vi "Configure Average.vi"(5 "Filter Count (10)":i32=10, 6 "Filter Mode (0: Repeat)":i32(ring) items=["Repeat", "Moving"], 7 "Filter Type (1: Scalar)":i32(ring)=1 items=["None", "Scalar", "Advanced"], 8 "error in (no error)":errorcluster, 9 "Enable Average Filter (F: Disable)":bool, 10 "Measurement Function (0: Voltage)":i32(ring) items=["Voltage", "Current", "Resistance", "Charge"], 11 "VISA resource name":refnum<visa-resource-name>) -> (0 "error out":errorcluster, 3 "VISA resource name out":refnum<visa-resource-name>)   [LabVIEW 2019, in "Keithley 6517.lvlib"]
doc: "Configures the average settings for the measurement functions (Voltage, Current, Resistance and Charge).\n\nNote:\nThe specified measurement should be enabled from <b>Configure Measurement Function.vi</b>.\n\nThis VI is <B>NOT</B> compatible with model <B>6514</B>."
uses:
  Keithley 6517.lvlib
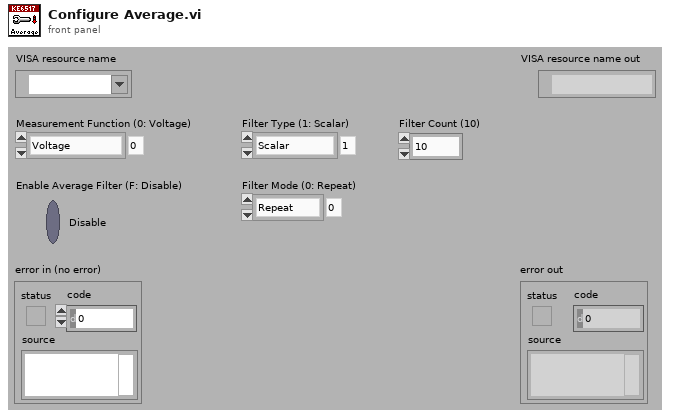
[diagram p1: front panel]
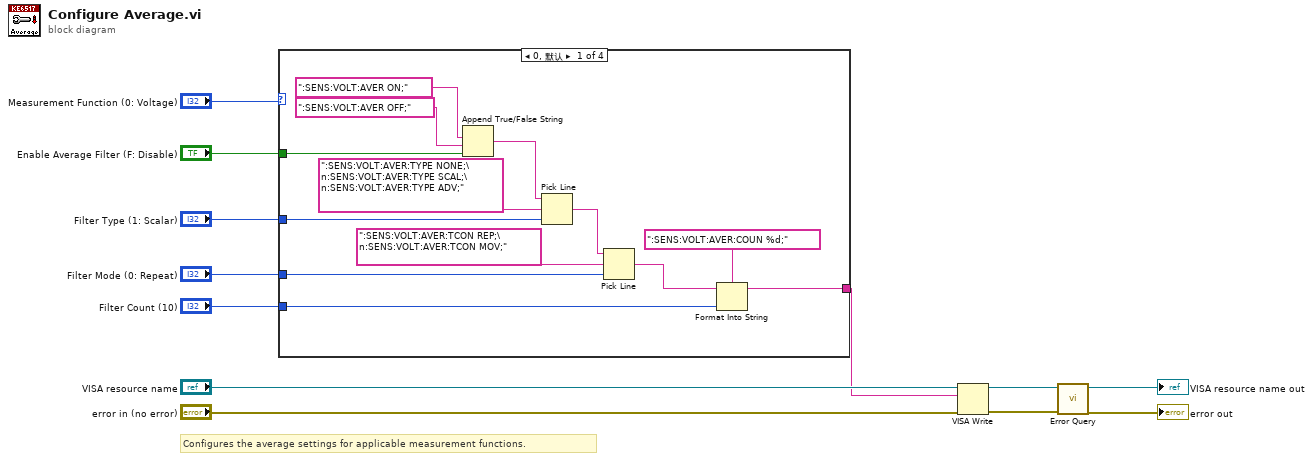
[diagram p0: block diagram]
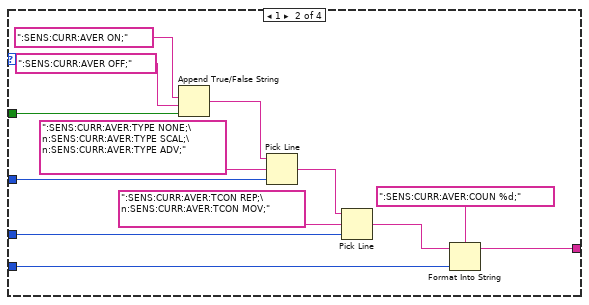
[diagram p2: hidden frame]
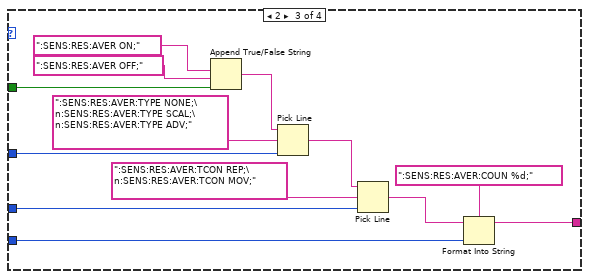
[diagram p3: hidden frame]
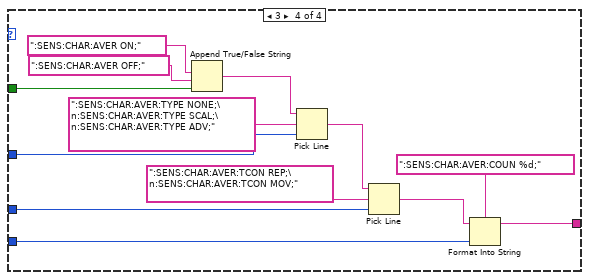
[diagram p4: hidden frame]
diagram:
  # "Configures the average settings for applicable measurement functions."
  n1 = case shown="0, 默认" "Measurement Function (0: Voltage)" {
    tunnel: "Enable Average Filter (F: Disable)" -> [w22 w35 w48 w61]
    tunnel: "Filter Type (1: Scalar)" -> [w19 w32 w45 w57]
    tunnel: "Filter Mode (0: Repeat)" -> [w16 w29 w44 w54]
    tunnel: "Filter Count (10)" -> [w15 w28 w40 w53]
    tunnel: [w13 w26 w39 w52] -> w3
    frame 0, Default {
      n2 = Append True/False String(1:w22, 2:":SENS:VOLT:AVER OFF;", 3:":SENS:VOLT:AVER ON;") -> (0:w20:string)  [unwired: 1 in]
      n3 = Pick Line(string ("")=w20, multi-line string=":SENS:VOLT:AVER:TYPE NONE;\n:SENS:VOLT:AVER:TYPE SCAL;\n:SENS:VOLT:AVER:TYPE ADV;", line index=w19) -> (output string=w18:string)
      n4 = Pick Line(string ("")=w18, multi-line string=":SENS:VOLT:AVER:TCON REP;\n:SENS:VOLT:AVER:TCON MOV;", line index=w16) -> (output string=w14:string)
      n5 = Format Into String(format string=":SENS:VOLT:AVER:COUN %d;", initial string=w14, w15) -> (resulting string=w13:string)  [unwired: 1 in, 1 out]
    }
    frame 1 {
      n6 = Append True/False String(1:w35, 2:":SENS:CURR:AVER OFF;", 3:":SENS:CURR:AVER ON;") -> (0:w34:string)  [unwired: 1 in]
      n7 = Pick Line(string ("")=w34, multi-line string=":SENS:CURR:AVER:TYPE NONE;\n:SENS:CURR:AVER:TYPE SCAL;\n:SENS:CURR:AVER:TYPE ADV;", line index=w32) -> (output string=w31:string)
      n8 = Pick Line(string ("")=w31, multi-line string=":SENS:CURR:AVER:TCON REP;\n:SENS:CURR:AVER:TCON MOV;", line index=w29) -> (output string=w27:string)
      n9 = Format Into String(format string=":SENS:CURR:AVER:COUN %d;", initial string=w27, w28) -> (resulting string=w26:string)  [unwired: 1 in, 1 out]
    }
    frame 2 {
      n10 = Append True/False String(1:w48, 2:":SENS:RES:AVER OFF;", 3:":SENS:RES:AVER ON;") -> (0:w47:string)  [unwired: 1 in]
      n11 = Pick Line(string ("")=w47, multi-line string=":SENS:RES:AVER:TYPE NONE;\n:SENS:RES:AVER:TYPE SCAL;\n:SENS:RES:AVER:TYPE ADV;", line index=w45) -> (output string=w42:string)
      n12 = Pick Line(string ("")=w42, multi-line string=":SENS:RES:AVER:TCON REP;\n:SENS:RES:AVER:TCON MOV;", line index=w44) -> (output string=w41:string)
      n13 = Format Into String(format string=":SENS:RES:AVER:COUN %d;", initial string=w41, w40) -> (resulting string=w39:string)  [unwired: 1 in, 1 out]
    }
    frame 3 {
      n14 = Append True/False String(1:w61, 2:":SENS:CHAR:AVER OFF;", 3:":SENS:CHAR:AVER ON;") -> (0:w59:string)  [unwired: 1 in]
      n15 = Pick Line(string ("")=w59, multi-line string=":SENS:CHAR:AVER:TYPE NONE;\n:SENS:CHAR:AVER:TYPE SCAL;\n:SENS:CHAR:AVER:TYPE ADV;", line index=w57) -> (output string=w55:string)
      n16 = Pick Line(string ("")=w55, multi-line string=":SENS:CHAR:AVER:TCON REP;\n:SENS:CHAR:AVER:TCON MOV;", line index=w54) -> (output string=w60:string)
      n17 = Format Into String(format string=":SENS:CHAR:AVER:COUN %d;", initial string=w60, w53) -> (resulting string=w52:string)  [unwired: 1 in, 1 out]
    }
  }
  n18 = VISA Write(VISA resource name="VISA resource name", write buffer=w3, error in (no error)="error in (no error)") -> (VISA resource name out=w11:refnum<visa-resource-name>, error out=w10:errorcluster)  [unwired: 1 out]
  n19 = call "Error Query.vi"("error in (no error)"=w10, "VISA resource name"=w11) -> ("error out"=→"error out":errorcluster, "VISA resource name out"=→"VISA resource name out":refnum<visa-resource-name>)  [unwired: 6 in, 2 out]
